vi "32xx_Decod_Local_Remote.vi"(11 "Réponse":string) -> (3 "Local/Remote":enum16{"Local", "Remote"}(ring))   [LabVIEW 2020]
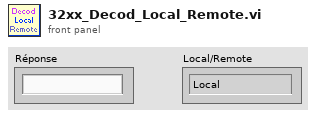
[diagram p1: front panel]
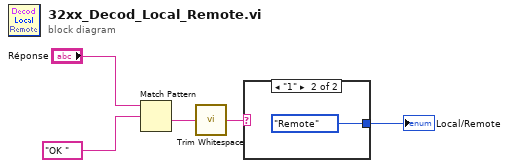
[diagram p0: block diagram]
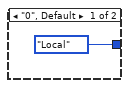
[diagram p2: hidden frame]
diagram:
  n1 = Match Pattern(string="Réponse", regular expression="OK " ("expression régulière")) -> (after substring=w5:string)  [unwired: 1 in, 3 out]
  n2 = call <vilib>:"Trim Whitespace.vi"("string"=w5) -> ("trimmed string"=w4:string)  [unwired: 1 in]
  n3 = case shown="\"1\"" w4 {
    tunnel: [enum16{"Local", "Remote"}."Local" ("Énum") enum16{"Local", "Remote"}."Remote" ("Énum")] -> w3
    frame "0", Default {
    }
    frame "1" {
    }
  }
  "Local/Remote" <- w3
